vi "DHE_GetDetXYSize.vi"() -> (7 "DHE_DetYsize":i32, 9 "DHE_DetXsize":i32)   [LabVIEW 2016]
uses:
  private/vis/DHE_GBLDriverVariables.vi
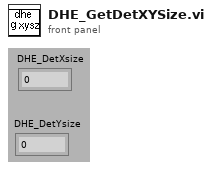
[diagram p1: front panel]
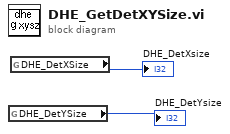
[diagram p0: block diagram]
diagram:
  n1 = global read "DHE_GBLDriverVariables.vi" "DHE_DetYSize"() -> (→"DHE_DetYsize":i32)
  n2 = global read "DHE_GBLDriverVariables.vi" "DHE_DetXSize"() -> (→"DHE_DetXsize":i32)
